vi "UT--Construct URIs.vi"() -> (3 "Test Passed?":bool)   [LabVIEW 2019]
doc: "JKI State Machine Objects (SMO) 1.3.0.56\nJKI - JKI\nCopyright (c) 2017, JKI"
uses:
  URI.lvlib
panel:
  out "Test Results":string[](array[string])
  out "Deconstructed URIs Under Test":T1={"protocols"=["opc.tcp", "opc.tcp", "", "", "opc.tcp", "", "opc.tcp", "http", "", "", "", "http", "sftp", "ni-rio", "my-own", "jki", "opc.tcp", "sftp", "", "", "http", "http"], "addresses"=["localhost", "localhost", "localhost", "localhost", "192.168.0.114", "192.168.0.114", "192.168.0.114", "192.168.0.11", "", "", "localhost", "192.168.0.11", "192.168.0.11", "192.168.0.8", "localhost", "169.254.244.4", "localhost", "192.168.0.11", "//192.168.0.101", "//192.168.0.101", "domain.com", "delicious.com"], "ports"=["49580", "49580", "49580", "49580", "49580", "49580", "49580", "", "", "", "80", "80", "22", "", "", "8080", "49580", "22", "", "", "", ""], "paths"=["", "Battery.AvailableEnergy", "Battery.AvailableEnergy", "Battery.AvailableEnergy", "Battery.Voltage", "Battery.Voltage", "Battery/data", "home2", "Battery/data", "Battery/data:TotalPowerRev (kW)", "Battery/data:TotalPowerRev (kW)", "Battery/data:TotalPowerRev (kW)", "home/lvuser", "", "Camera/FrameRate", "SuperSecretPrivateStuff/value", "", "home/lvuser/", "EnergyCell", "/EnergyCell", "function.cgi", "post"], "Arguments"=[{"Arguments"=[]}, {"Arguments"=[]}, {"Arguments"=[]}, {"Arguments"=[]}, {"Arguments"=[]}, {"Arguments"=[]}, {"Arguments"=[]}, {"Arguments"=[]}, {"Arguments"=[]}, {"Arguments"=[]}, {"Arguments"=[]}, {"Arguments"=[]}, {"Arguments"=[]}, {"Arguments"=[]}, {"Arguments"=[]}, {"Arguments"=[]}, {"Arguments"=[]}, {"Arguments"=[]}, {"Arguments"=[]}, {"Arguments"=[]}, {"Arguments"=[{"key"="url", "value"="http://fonzi.com/"}, {"key"="name", "value"="Fonzi"}, {"key"="mood", "value"="happy"}, {"key"="coat", "value"="leather"}]}, {"Arguments"=[{"key"="url", "value"="http://domain.tld/"}, {"key"="title", "value"="The title of a post"}]}]}
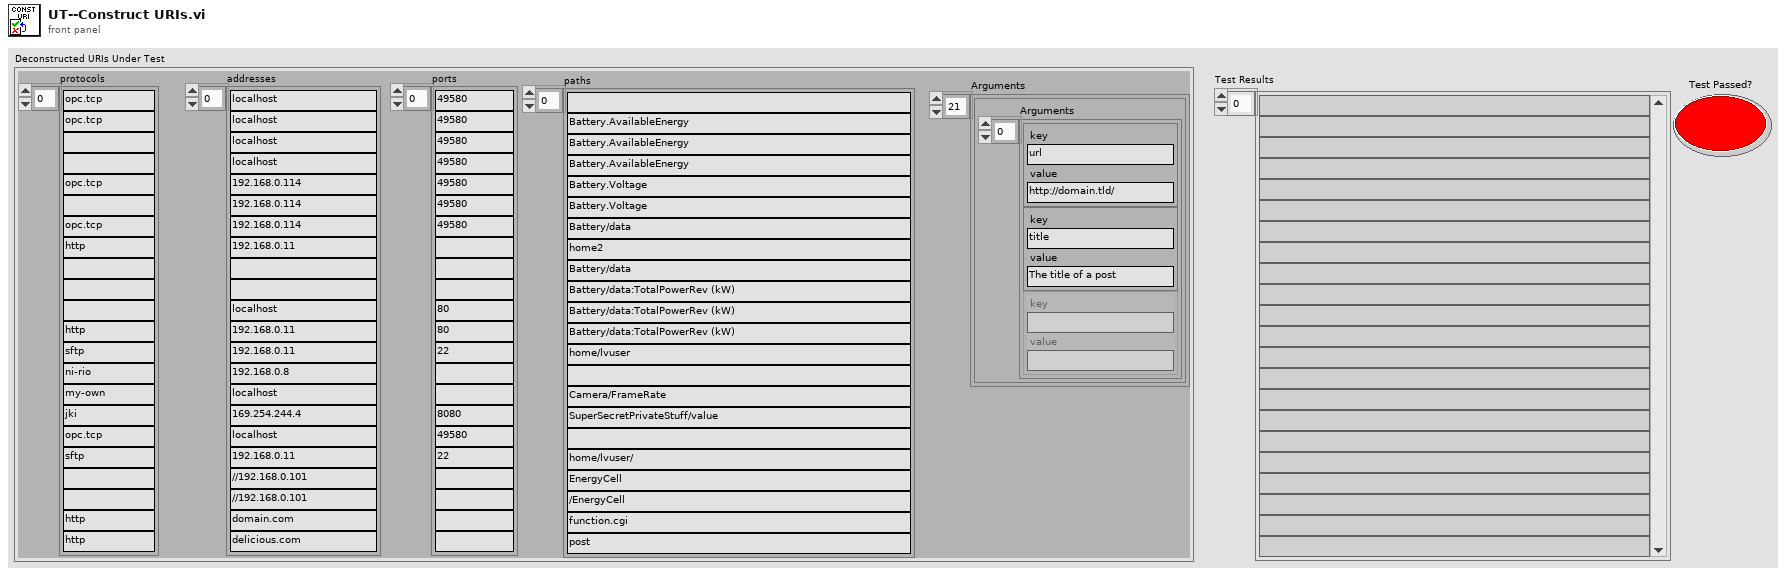
[diagram p1: front panel]
types:
  T1 = cluster{"protocols":string[], "addresses":string[], "ports":string[], "paths":string[], "Arguments":cluster{"Arguments":cluster{"key":string, "value":string}[]}[]}
  T2 = cluster{"Arguments":cluster{"key":string, "value":string}[]}[]
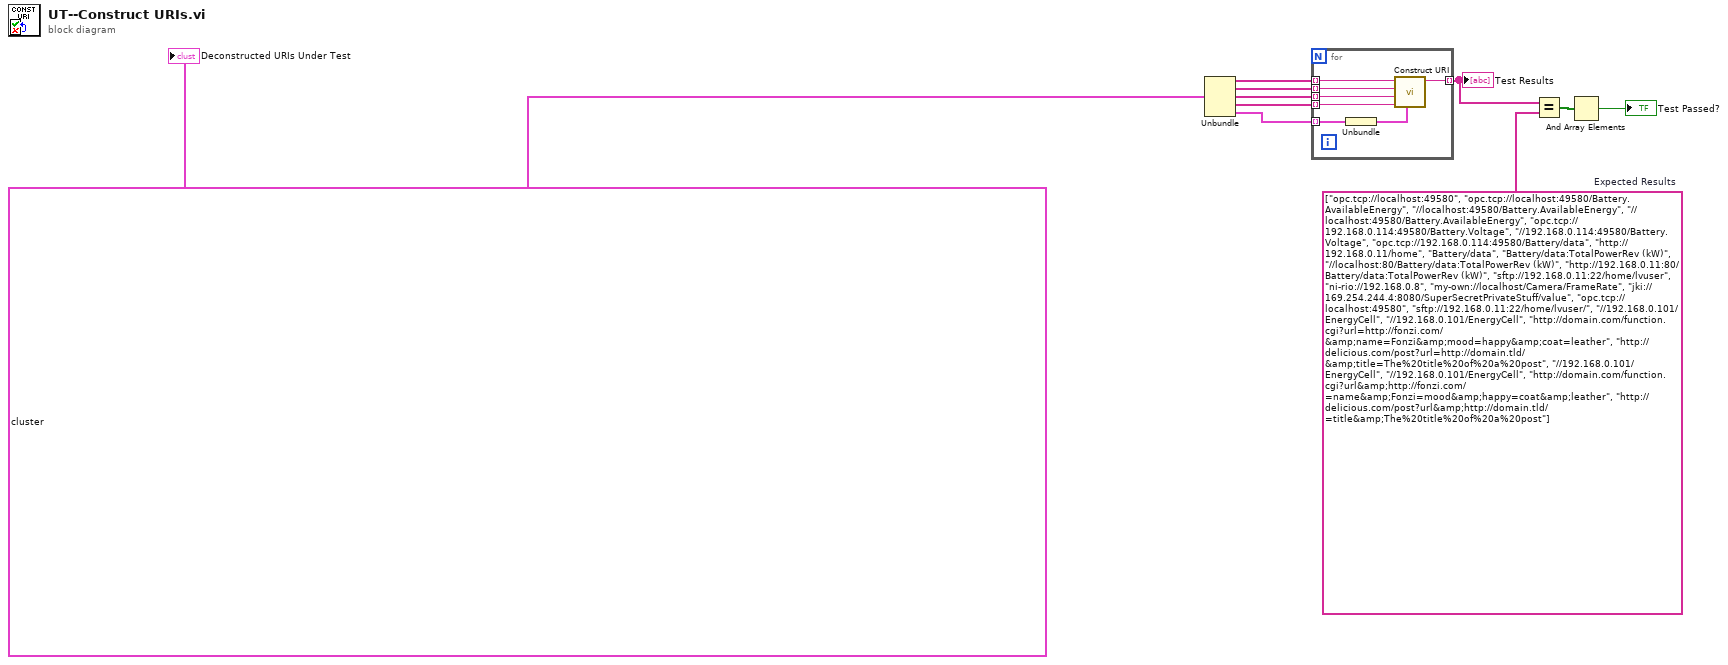
[diagram p0: block diagram]
diagram:
  w3 = string[] ["opc.tcp://localhost:49580", "opc.tcp://localhost:49580/Battery.AvailableEnergy", "//localhost:49580/Battery.AvailableEnergy", "//localhost:49580/Battery.AvailableEnergy", "opc.tcp://192.168.0.114:49580/Battery.Voltage", "//192.168.0.114:49580/Battery.Voltage", "opc.tcp://192.168.0.114:49580/Battery/data", "http://192.168.0.11/home", "Battery/data", "Battery/data:TotalPowerRev (kW)", "//localhost:80/Battery/data:TotalPowerRev (kW)", "http://192.168.0.11:80/Battery/data:TotalPowerRev (kW)", "sftp://192.168.0.11:22/home/lvuser", "ni-rio://192.168.0.8", "my-own://localhost/Camera/FrameRate", "jki://169.254.244.4:8080/SuperSecretPrivateStuff/value", "opc.tcp://localhost:49580", "sftp://192.168.0.11:22/home/lvuser/", "//192.168.0.101/EnergyCell", "//192.168.0.101/EnergyCell", "http://domain.com/function.cgi?url=http://fonzi.com/&amp;name=Fonzi&amp;mood=happy&amp;coat=leather", "http://delicious.com/post?url=http://domain.tld/&amp;title=The%20title%20of%20a%20post", "//192.168.0.101/EnergyCell", "//192.168.0.101/EnergyCell", "http://domain.com/function.cgi?url&amp;http://fonzi.com/=name&amp;Fonzi=mood&amp;happy=coat&amp;leather", "http://delicious.com/post?url&amp;http://domain.tld/=title&amp;The%20title%20of%20a%20post"]  # Expected Results
  w10 = T1 {"protocols"=["opc.tcp", "opc.tcp", "", "", "opc.tcp", "", "opc.tcp", "http", "", "", "", "http", "sftp", "ni-rio", "my-own", "jki", "opc.tcp", "sftp", "", "", "http", "http"], "addresses"=["localhost", "localhost", "localhost", "localhost", "192.168.0.114", "192.168.0.114", "192.168.0.114", "192.168.0.11", "", "", "localhost", "192.168.0.11", "192.168.0.11", "192.168.0.8", "localhost", "169.254.244.4", "localhost", "192.168.0.11", "//192.168.0.101", "//192.168.0.101", "domain.com", "delicious.com"], "ports"=["49580", "49580", "49580", "49580", "49580", "49580", "49580", "", "", "", "80", "80", "22", "", "", "8080", "49580", "22", "", "", "", ""], "paths"=["", "Battery.AvailableEnergy", "Battery.AvailableEnergy", "Battery.AvailableEnergy", "Battery.Voltage", "Battery.Voltage", "Battery/data", "home", "Battery/data", "Battery/data:TotalPowerRev (kW)", "Battery/data:TotalPowerRev (kW)", "Battery/data:TotalPowerRev (kW)", "home/lvuser", "", "Camera/FrameRate", "SuperSecretPrivateStuff/value", "", "home/lvuser/", "EnergyCell", "/EnergyCell", "function.cgi", "post"], "Arguments"=[{"Arguments"=[]}, {"Arguments"=[]}, {"Arguments"=[]}, {"Arguments"=[]}, {"Arguments"=[]}, {"Arguments"=[]}, {"Arguments"=[]}, {"Arguments"=[]}, {"Arguments"=[]}, {"Arguments"=[]}, {"Arguments"=[]}, {"Arguments"=[]}, {"Arguments"=[]}, {"Arguments"=[]}, {"Arguments"=[]}, {"Arguments"=[]}, {"Arguments"=[]}, {"Arguments"=[]}, {"Arguments"=[]}, {"Arguments"=[]}, {"Arguments"=[{"key"="url", "value"="http://fonzi.com/"}, {"key"="name", "value"="Fonzi"}, {"key"="mood", "value"="happy"}, {"key"="coat", "value"="leather"}]}, {"Arguments"=[{"key"="url", "value"="http://domain.tld/"}, {"key"="title", "value"="The title of a post"}]}]} ("Test Results")
  n1 = Unbundle(w10) -> ("protocols"=w9:string[], "addresses"=w8:string[], "ports"=w7:string[], "paths"=w6:string[], "Arguments"=w5:T2)
  n2 = for {
    tunnel: w9 -> [w17] mode=indexing
    tunnel: w8 -> [w16] mode=indexing
    tunnel: w7 -> [w15] mode=indexing
    tunnel: w6 -> [w14] mode=indexing
    tunnel: [w13] -> w4 mode=indexing
    tunnel: w5 -> [w12] mode=indexing
    n3 = Unbundle(w12) -> ("Arguments"=w11:cluster{"key":string, "value":string}[])
    n4 = call "Construct URI.vi"("Arguments"=w11, "path"=w14, "port"=w15, "address"=w16, "protocol"=w17) -> ("URI"=w13:string)  [unwired: 6 in]
  }
  "Test Results" <- w4
  n5 = Equal?(x=w4, y=w3) -> (x = y?=w2:bool[])
  n6 = And Array Elements(Boolean array=w2) -> (logical AND=→"Test Passed?":bool)
  "Deconstructed URIs Under Test" <- w10
